vi "HFRR ADV v13.vi"() -> ()   [LabVIEW 2025] (continued)
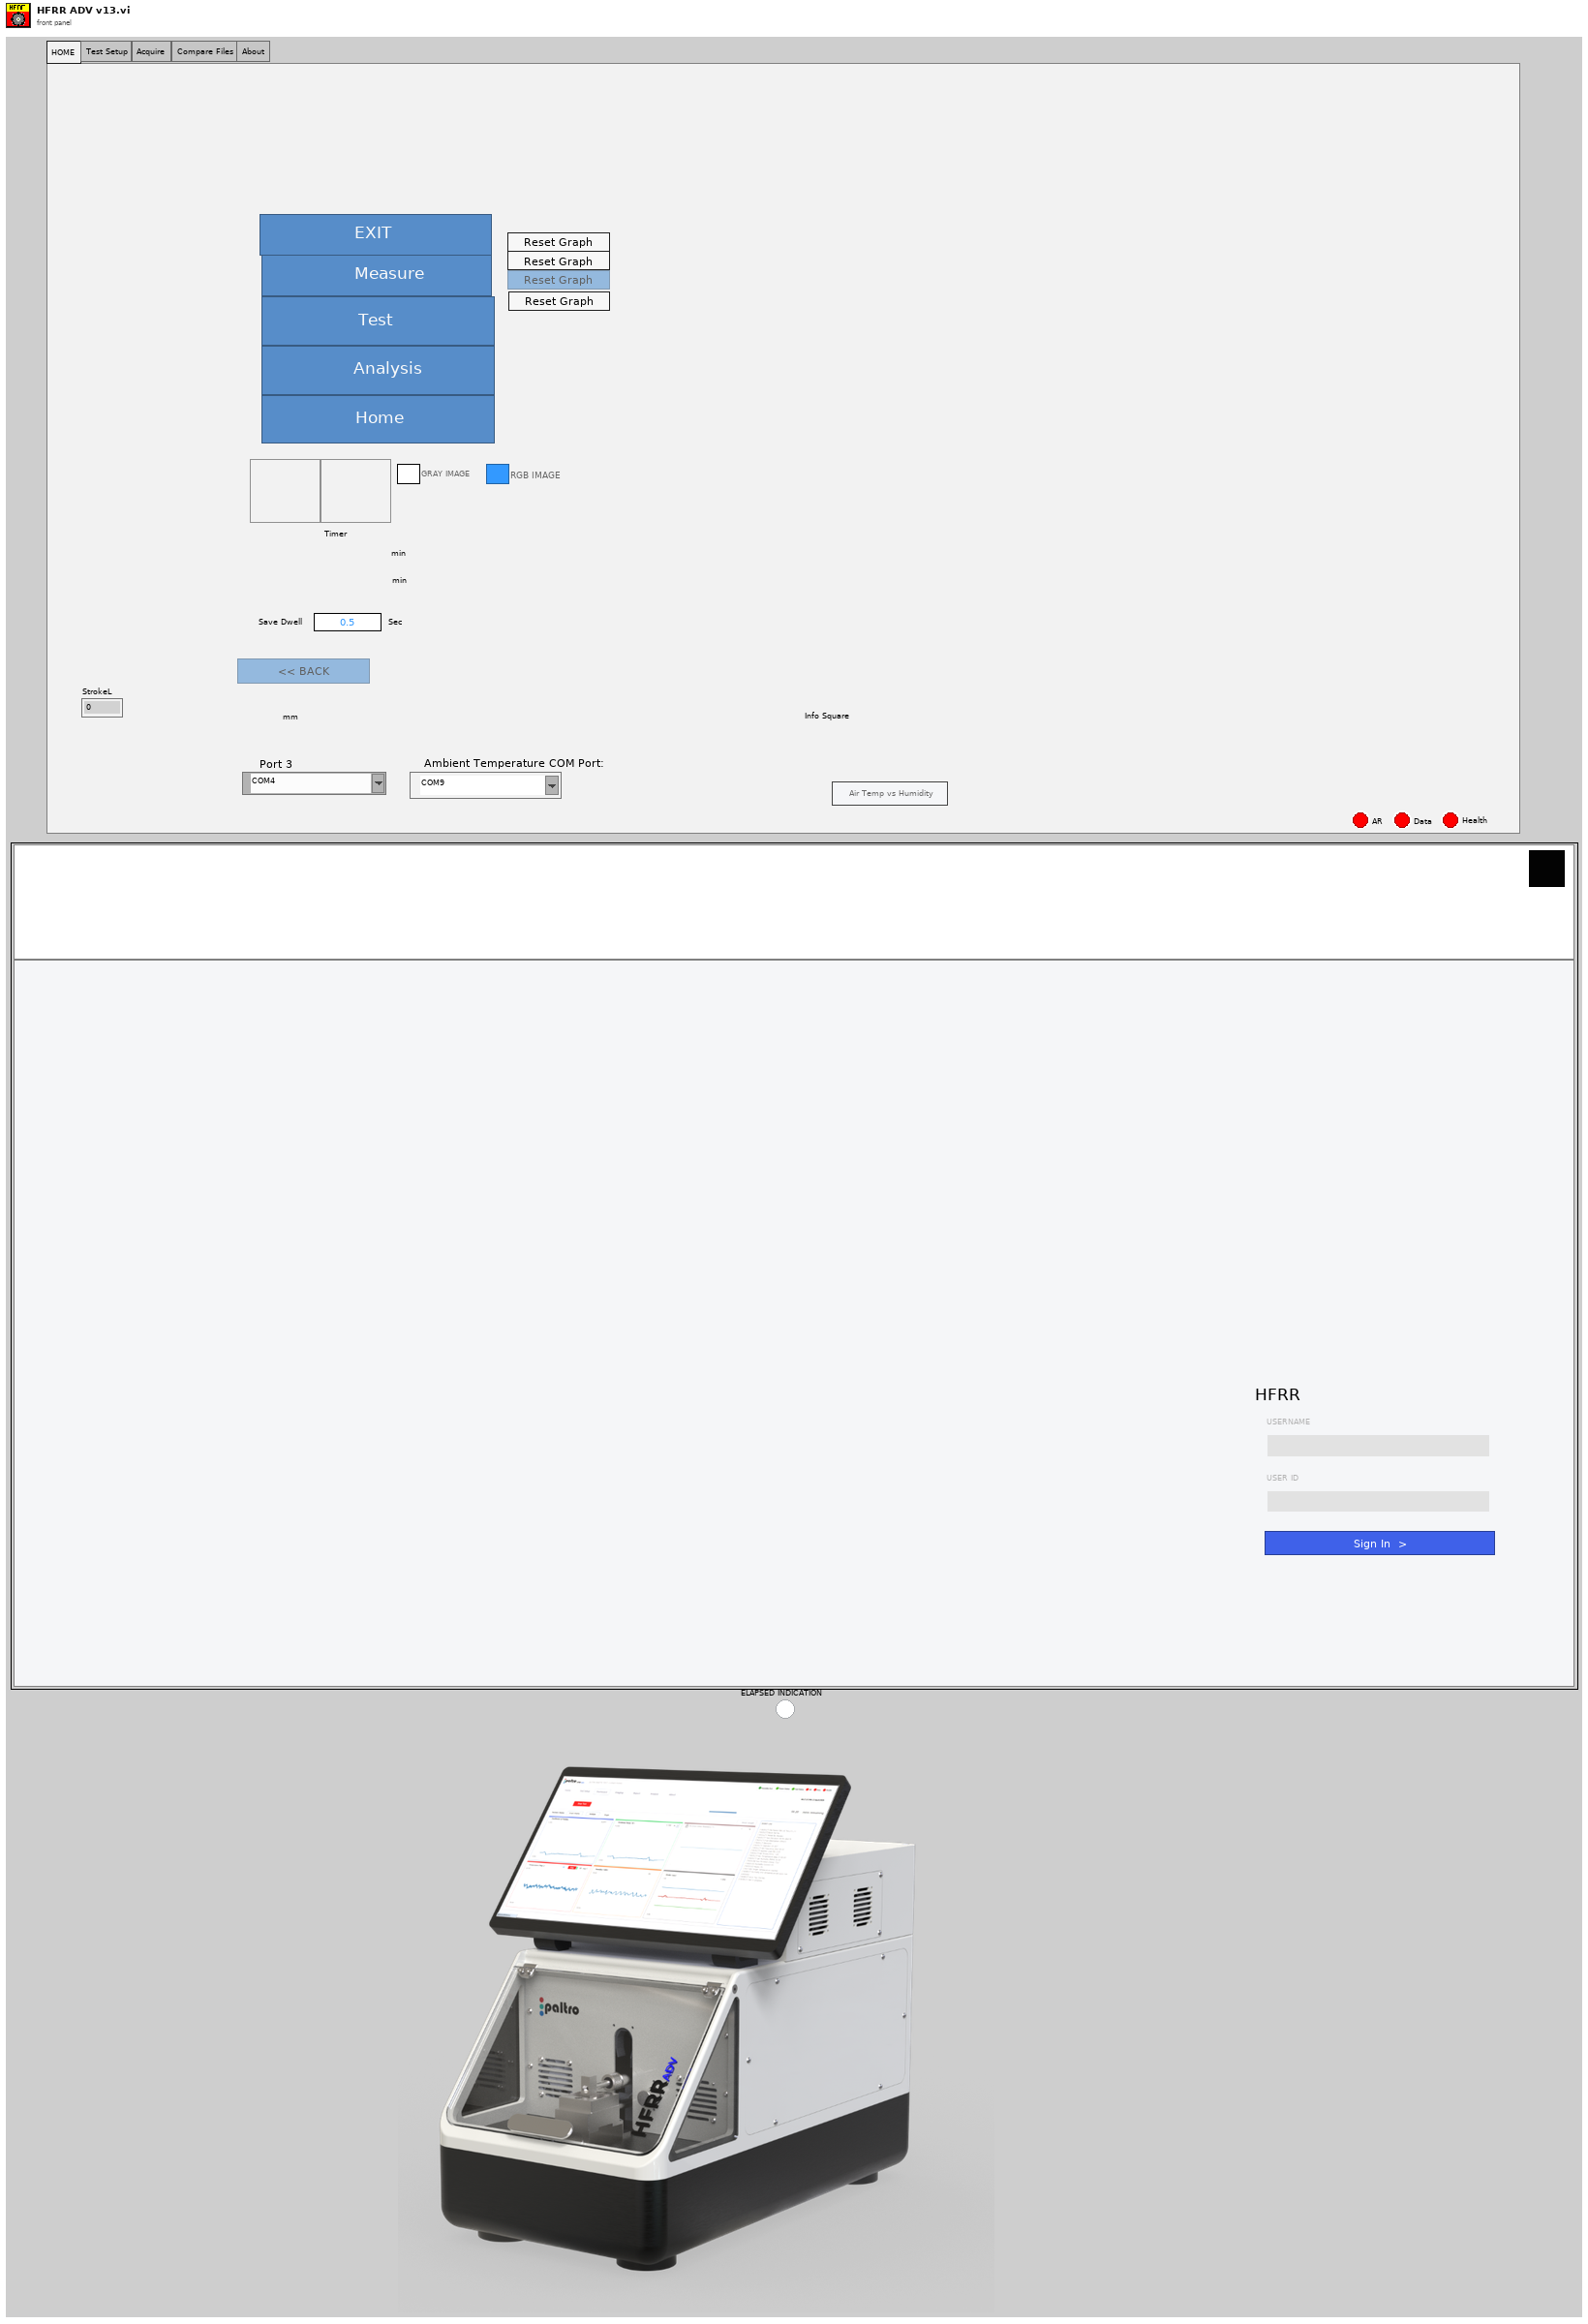
[diagram p1: front panel]
types:
  T1 = enum32{"Home", "Dashboard", "Imaging", "Report", "Analysis", "About", "Test Setup", "Advance"}
  T2 = enum32{"HOME", "Test Setup", "Acquire", "Adv Scar", "Adv Scar Report", "Compare Files", "About", "Advance", "Mooha"}
  T3 = enum16{"ASTM D6079", "ISO 12156", "CEC F-096-A-06", "Custom"}
  T4 = enum32{"Dashboard 1", "Dashboard 2", "Dashboard 3"}
  T5 = enum32{"COF", "Friction", "ECR", "Temperature", "Humidity", "Stroke"}
  T6 = enum32{"Coefficient Of Friction", "Air Temperature", "Humidity", "Stroke", "Sample Temperature", "Electrical Contact Resistance", "Frequency", "Air Temp vs Rh"}
  T7 = enum32{"Gains", "Configuration Parameters", "Temperature Calibration"}
  T8 = enum32{"Stroke Data", "Temperature Calibration", "Friction Force Raw Data"}
  T9 = cluster{"Proportional Gain (Kc)":dbl, "Integral Time (Ti, min)":dbl, "Derivative Time (Td, min)":dbl}
  T10 = enum32{"Temp Variables", "Camera", "WO 2465 (1)", "WO 2465 (2)", "WO 2465 (3)"}
  T11 = typedef "Auto Start enum.ctl" = enum16{"Init", "Humidity & Temperature On", "Reach point", "Maintain Stage", "Start Stage", "close", "Exit"}
  T12 = enum32{"Freqz control", "Low Speed Analog Inputs & Digital IOs", "Temperature Tuning", "Voltage LVDT raw", "High Speed Analog Inputs - Displacement & Friction", "LVDT Calibration", "Sericve", "Friction Force Calibration", "Bytes At Port", "Loadcell Board"}
  T13 = cluster{"proportional gain (Kc)":dbl, "integral time (Ti, min)":dbl, "derivative time (Td, min)":dbl}
  T14 = typedef "imagedata.ctl" = cluster{"image type":i32, "image depth":i32, "image":u8[], "mask":u8[], "colors":u32[], "Rectangle":cluster{"left":i16, "top":i16, "right":i16, "bottom":i16}}
  T15 = enum32{"HOME", "Test Setup", "Acquire", "Compare Files", "Print Report", "About", "Advance", "Mooha"}
  T16 = enum8{"Enabled", "Disabled", "Disabled and Grayed Out"}
  T17 = cluster{"Read Heave and Surge":string, "Bytes at Heave Port":dbl, "Heave and Surge COM Port:":refnum<visa-resource-name>, "Com Port 2":refnum<visa-resource-name>, "Residual Due":string, "Heave COM Status 2":bool, "Heave COM Status":bool, "Port 2":bool, "Sway PPR":dbl, "Surge PPR":dbl, "Heave PPR":dbl, "Sway Pitch":dbl, "Surge Pitch":dbl, "Heave Pitch":dbl, "Sway Pulses/mm":dbl, "Surge Pulses/mm":dbl, "Heave Pulses/mm":dbl, "inner loop":dbl, "Read Heave and Surge 2":string, "String 36":string, "Write S":bool, "WriteCC1":string[], "Heave COM Loop":i32, "LastCom":string, "EXIT":bool, "Error Heave":errorcluster}
  T18 = enum16{"Always On", "Always Off", "Off While Running"}
  T19 = typedef "POST ANALYSIS ENUM.ctl" = enum16{"OPEN EXE", "INIT", "OPEN FILE", "FIT", "DRAW REC", "DRAW LINE", "PAN", "ZOOM IN", "ZOOM OUT", "SET ZOOM", "CLEAR ROI", "GET MEASUREMENTS", "RESIZE MODE", "STREAM START", "STREAM STOP", "SHOW UI", "MINIMIZE UI", "HIDE UI", "CKISE APP", "CLOSE CONNECTION", "SAVE IMAGE", "SET ROI COLOR", "READ", "TCP CHECK", "CLOSE"}
  T20 = typedef "CAMERA LIVE FEED ENUM.ctl" = enum16{"OPEN EXE", "INIT", "READ", "CAMERA CONNECT", "CAMERA START", "CAMERA STOP", "CAMERA GRAY", "CAMERA RGB", "CAMERA MINIMIZE", "CAMERA CLOSE", "CAMERA MODE LIST", "CAMERA MODE SET", "CAMERA RESTORE", "CAMERA SAVE", "CLOSE"}
  T21 = cluster{"File Name":string, "Test Method":string, "Operator":string, "Fuel Description":string, "Date and time":string}
  T22 = enum32{"Home", "Dashboard", "Imaging", "Report", "Analysis", "About", "Test Setup"}
  T23 = enum32{"HOME", "Test Setup", "Acquire", "Compare Files", "About", "Advance", "Mooha"}
  T24 = enum16{"deny read/write", "deny write-only", "deny none"}
  T25 = typedef "NI_ReportGenerationCore.lvlib/HTML Report Image Alignment.ctl" = enum16{"(default)", "LEFT", "RIGHT", "TOP", "TEXTTOP", "MIDDLE", "ABSMIDDLE", "BASELINE", "BOTTOM", "ABSBOTTOM"}
  T26 = enum16{"open", "replace", "create", "open or create", "replace or create", "replace or create with confirmation"}
  T27 = enum16{"INIT", "READ", "MANUAL WRITE", "WRITE", "CLOSE", "ERROR INIT"}
  T28 = enum16{"open", "open or create", "create or replace", "create", "open (read only)"}
  T29 = cluster{"Mode":enum16{"RTU", "ASCII"}, "Slave Address":u8}
diagram:
  w5 = FALSE ("Visible")
  w6 = T16."Enabled" ("Disabled")
  w9 = FALSE ("Visible")
  w8 = FALSE ("Humidity Off Command")
  w28 = "" ("USER ID")
  # "[CH1]    - FF\n[CH2]   - TEMPERATURE\n[CH3]    - Humidity\n[CH4]    - AIR TEMP\n[CH5]\\- Visa Uno\n[CH6] \\- Visa Due\n[CH7]  \\- file path\n[CH8]   - Displacement Gain\n[CHA]   - Stroke Gain\n[CHB]   - Stroke PID Gain\n[CHC]   -Language Selection\n[CHD]   -Power +\n[CHE]   -Power_\n[CHF]   -Heater\n[CHG]   -Humidity Wet\n[CHH]   -Humidity Dry\n[CHI]   -Integral Time \n[CHIJ   -Air intercept\n[CHI]   -Temp Intercept"
  n1 = flat-sequence {
    tunnel: [w83] -> w19
    tunnel: w19 -> [w97]
    tunnel: [w96] -> w18
    tunnel: ["ao0"] -> w21
    tunnel: w18 -> [_]
    tunnel: w21 -> [w162]
    tunnel: [w162] -> w20
    tunnel: w20 -> [w215]
    tunnel: [w213] -> w32
    tunnel: [w215] -> w31
    tunnel: w32 -> [w266]
    tunnel: w31 -> [w222]
    tunnel: [w266] -> w17
    tunnel: [w228] -> w16
    tunnel: [w216] -> w15
    tunnel: [w273] -> _
    tunnel: [w272] -> _
    tunnel: [w274] -> w60
    tunnel: w17 -> [w274]
    tunnel: w16 -> [w272]
    tunnel: w15 -> [w273]
    frame #0 {
      n2 = control-ref of="This VI"() -> (w71:refnum<vi>)
      n3 = property class="VI"(reference=w71) -> (reference out=w62:refnum<vi>, error out=w66:errorcluster, "Panel"=w70:refnum<vi>)  [unwired: 1 in]
      n4 = property class="Pnl"(reference=w70, error in=w66) -> (reference out=w64:refnum<vi>, error out=w67:errorcluster, "Panes[]"=w69:refnum<vi>[])
      n5 = for {
        tunnel: w69 -> [w77] mode=indexing
        tunnel: T18."Always Off" ("Horizontal Scrollbar Visibility") -> [w76]
        tunnel: w67 -> [w73]
        tunnel: [w72] -> w65
        n6 = property class="Pane"(reference=w77, error in=w73, "HorizScrollbarVisibility"=w76) -> (reference out=w74:refnum<vi>, error out=w75:errorcluster)
        n7 = Close Reference(reference=w74, error in (no error)=w75) -> (error out=w72:errorcluster)
      }
      n8 = Close Reference(reference=w64, error in (no error)=w65) -> (error out=w63:errorcluster)
      n9 = Close Reference(reference=w62, error in (no error)=w63) -> (error out=→"error out 8":errorcluster)
    }
    frame #1 {
      n10 = call "CLOSE CONNECTION.vi"("error in (no error)"="error in (no error) 2") -> ("error out"=w81:errorcluster)  [unwired: 10 in]
      n11 = call <vilib>:"Clear Errors.vi"("error in (no error)"=w81) -> ("error out"=w80:errorcluster)  [unwired: 5 in, 1 out]
      n12 = disable-structure shown="Enabled" {
        disable-tunnel: w80 -> [w87 _]
        disable-tunnel: [w86 _] -> w83
        frame Enabled {
          n13 = call <userlib>:"Fit VI window to Largest Dec.vi"("error in (no error)"=w87, "border spacing (2 px)"=1) -> ("error out"=w90:errorcluster, "dup VI Ref"=w94:refnum<vi>)  [unwired: 4 in]
          n14 = invoke on="Invoke Node" class="VI" method="FP.Run-Time Position.Maximized"(reference=w94, error in=w90) -> (error out=w91:errorcluster)  [unwired: 2 in, 3 out]
          n15 = call <vilib>:"Clear Errors.vi"("error in (no error)"=w91) -> ("error out"=w93:errorcluster)  [unwired: 5 in, 1 out]
          n16 = control-ref of="This VI"() -> (w85:refnum<vi>)
          n17 = invoke on="Invoke Node" class="VI" method="Default Vals.Reinit All"(reference=w85, error in=w93) -> (reference out=w89:refnum<vi>, error out=w88:errorcluster)  [unwired: 1 in, 1 out]
          n18 = Close Reference(reference=w89, error in (no error)=w88) -> (error out=w86:errorcluster)
        }
        frame Disabled {
        }
      }
      n19 = local write "sign in temp"(FALSE ("sign in temp")) -> ()
      n20 = property on="Sign In" class="Bool (strict)"("DisabledEnum"=T16."Disabled" ("Disabled")) -> ()  [unwired: 2 in, 2 out]
      n21 = property on="Auto Scar Check" class="Clust (strict)"("Visible"=TRUE) -> ()  [unwired: 2 in, 2 out]
    }
    frame #2 {
      n22 = call "dialog box.vi"("Status"="Before starting the test, verify that the microscope cable is connected.", "error in"=w97) -> ("error out"=w96:errorcluster)  [unwired: 8 in]
    }
    frame #3 {
      w104 = FALSE ("Upld AR 2")
      # "kkkkk"
      # "C:\\Windows\\wndcm_pw_stdED hfrr.txt"
      # "C:\\LAB-IQ NXT"
      # "C:\\LAB-IQ NXT\\wndcm_pw_stdED hfrr.txt"
      # "password file"
      n23 = Current VI's Path() -> (path=w117:path)
      n24 = Strip Path(path=w117) -> (stripped path=w110:path)  [unwired: 1 out]
      n25 = Path To String(path=w110) -> (string=w112:string)
      n26 = local write "conststatus"(0.0 ("rpm value : 2")) -> ()
      n27 = local write "Upld AR 2"(TRUE ("Upld AR 2")) -> ()
      n28 = local write "Lan flag"(0.0 ("Lan flag")) -> ()
      n29 = local write "COUNT"(0 ("COUNT")) -> ()
      n30 = local write "FLAG 2"(0.0 ("FLAG 2")) -> ()
      n31 = local write "Com flag"(u32 0 ("Com flag")) -> ()
      n32 = local write "Re-Initialise"(TRUE ("Re-Initialise")) -> ()
      n33 = local write "refresh flag"(FALSE ("refresh flag")) -> ()
      n34 = local write "Json St Flg"(w104) -> ()
      n35 = Search/Split String(string=w112, search string/char (-)=".exe") -> (match + rest of string=w114:string)  [unwired: 1 in, 2 out]
      n36 = Match True/False String(2:".vi" ("false string"), 3:".exe" ("true string"), 4:w114) -> (0:w111:bool)  [unwired: 1 out]
      n37 = local write "Json End Flg"(w104) -> ()
      n38 = case shown="True" w111 {
        tunnel: w110 -> [w133 w135]
        tunnel: [w133 w134] -> w108
        frame False {
        }
        frame True {
          n39 = Strip Path(path=w135) -> (stripped path=w134:path)  [unwired: 1 out]
        }
      }
      n40 = Path To String(path=w108) -> (string=→"Gain path":string)
      n41 = local write "Main Tab Display"(T4."Dashboard 1" ("Main Tab Display")) -> ()
      n42 = local write "main tab sub"(enum32{"Page 1", "Page 2"}."Page 1" ("main tab sub")) -> ()
      n43 = local write "Main Tab"(T2."HOME" ("Main Tab")) -> ()
      n44 = local write "EVENT LOG"("") -> ()
      n45 = List Folder(path=path "C:/LAB-IQ" ("directory path"), pattern="*.txt") -> (filenames=w123:string[])  [unwired: 2 in, 3 out]
      n46 = Search 1D Array(1D array=w123, element="wndcm_pw_stdED hfrr.txt") -> (index of element=w126:i32)  [unwired: 1 in]
      n47 = Equal?(x=w126, y=-1) -> (x = y?=w121:bool)
      n48 = case shown="True" w121 {
        frame False {
        }
        frame True {
          n49 = String To Byte Array(string="123\n") -> (unsigned byte array=w140:u8[])
          n50 = Array Size(array=w140) -> (size(s)=w139:i32)
          n51 = for {
            N: w139 -> [_]
            tunnel: w140 -> [w153]
            tunnel: [w150] -> w142 mode=indexing
            tunnel: w139 -> [w145]
            i -> [w143]
            n52 = Decrement(x=w145) -> (x-1=w146:i32)
            n53 = Equal?(x=w143, y=w146) -> (x = y?=w147:bool)
            n54 = Index Array(array=w153, index=w143) -> (element=w152:u8)
            n55 = Number To Decimal String(number=w152) -> (decimal integer string=w151:string)  [unwired: 1 in]
            n56 = Select(t="", s=w147, f="\r") -> (s? t:f=w144:string)
            n57 = Concatenate Strings(w151, w144) -> (w150:string)
          }
          n58 = local read "file path"() -> (w136:path)
          n59 = Concatenate Strings(w142) -> (w138:string)
          n60 = call <vilib>:"Write Characters To File.vi"("append to file? (new file:F)"=FALSE, "character string"=w138, "file path (dialog if empty)"=w136) -> ()  [unwired: 2 in, 1 out]
        }
      }
      n61 = local write "clk"(0.0 ("clk")) -> ()
      n62 = local write "Flag"(0.0 ("Flag")) -> ()
      "file path" <- path "C:/LAB-IQ/wndcm_pw_stdED hfrr.txt" ("file path")
      "FF buffer" <- dbl[] [] ("FF buffer")
    }
    frame #4 {
      # "C:\\WinDucom\\calibrate WO 2391.dcf"
      n63 = String To Path(string="C:\\LAB-IQ\\calibrate WO 2465.dcf") -> (path=w161:path)
      n64 = Open/Create/Replace File "Open File"(file path (use dialog)=w161) -> (refnum out=w160:refnum<file>)  [unwired: 5 in, 2 out]
      n65 = for {
        N: 24 -> [_]
        tunnel: w160 -> [w181]
        i -> [w175]
        (unwired) TRUE ("line mode (F)")
        n66 = Read from Text File "Read File"(file (use dialog)=w181) -> (text=w180:string)  [unwired: 3 in, 3 out]
        n67 = Match Pattern(string=w180, regular expression="]") -> (after substring=w178:string)  [unwired: 1 in, 3 out]
        n68 = String Subset(string=w180, offset (0)=5, length (rest)=10 ("length (rest)")) -> (substring=w173:string)
        n69 = Fract/Exp String To Number(string=w173) -> (number=w174:dbl)  [unwired: 3 in, 1 out]
        n70 = Match Pattern(string=w178, regular expression="-") -> (before substring=w176:string)  [unwired: 1 in, 3 out]
        n71 = case shown="7" w175 {
          tunnel: w174 -> [w184 w185 w186 w187 _ _ _ w192 w193 w194 w197 w198 w199 w200 w201 w202 w203 w206 w207 _ _ w210 _ _ _]
          tunnel: w176 -> [_ _ _ _ w188 w189 w190 _ _ _ _ _ _ _ _ _ _ _ _ w208 w209 _ w211 w212 _]
          frame 0 {
            n72 = local write "FRIC. FORCE :"(w184) -> ()
          }
          frame 1 {
            n73 = local write "TEMPERATURE :"(w185) -> ()
          }
          frame 2 {
            n74 = local write "HUMIDITY:"(w186) -> ()
          }
          frame 3 {
            n75 = local write "AIR TEMPERATURE :"(w187) -> ()
          }
          frame 4 {
            n76 = local write "Com Port 1"(w188) -> ()
          }
          frame 5 {
            n77 = local write "Com Port 2"(w189) -> ()
            n78 = local write "visa due"(w189) -> ()
          }
          frame 6 {
            n79 = String To Path(string=w190) -> (path=w191:path)
            n80 = local write "File Path"(w191) -> ()
          }
          frame 7 {
            n81 = local write "DISPLACEMENT :"(w192) -> ()
          }
          frame 8 {
            n82 = local write "STROKE GAIN :"(w193) -> ()
          }
          frame 9 {
            n83 = local read "Stroke PID Gains"() -> (w196:T9)
            n84 = Bundle By Name(cluster=w196, "Proportional Gain (Kc)"=w194) -> (w195:T9)
            n85 = local write "Stroke PID Gains"(w195) -> ()
          }
          frame 10 {
            n86 = local write "Language Selection"(w197) -> ()
          }
          frame 11 {
            n87 = local write "CH-POWER +"(w198) -> ()
          }
          frame 12 {
            n88 = local write "CH-POWER -"(w199) -> ()
          }
          frame 13 {
            n89 = local write "CH-HEATER"(w200) -> ()
          }
          frame 14 {
            n90 = local write "CH-HUMIDITY WET"(w201) -> ()
          }
          frame 15 {
            n91 = local write "CH-HUMIDITY DRY"(w202) -> ()
          }
          frame 16 {
            n92 = local read "Stroke PID Gains"() -> (w205:T9)
            n93 = Bundle By Name(cluster=w205, "Integral Time (Ti, min)"=w203) -> (w204:T9)
            n94 = local write "Stroke PID Gains"(w204) -> ()
          }
          frame 17 {
            n95 = local write "AIR TEMP INTERCEPT:"(w206) -> ()
          }
          frame 18 {
            n96 = local write "TEMP INTERCEPT:"(w207) -> ()
          }
          frame 19 {
            n97 = local write "S.NO"(w208) -> ()
          }
          frame 20 {
            n98 = local write "Com Port 3"(w209) -> ()
          }
          frame 21 {
            n99 = local write "LvdtOff"(w210) -> ()
          }
          frame 22 {
            n100 = local write "C3 :"(w211) -> ()
          }
          frame 23 {
            n101 = local write "Camera Port :"(w212) -> ()
          }
          frame 24, Default {
          }
        }
      }
      n102 = String To Path(string="C:\\LAB-IQ\\Image Calibrate v01.dcf") -> (path=w157:path)
      n103 = Open/Create/Replace File ("Open File")(file path (use dialog)=w157) -> (refnum out=w156:refnum<file>)  [unwired: 5 in, 2 out]
      n104 = for {
        N: 4 -> [_]
        tunnel: w156 -> [w168]
        i -> [w164]
        n105 = Read from Text File ("Read File")(file (use dialog)=w168) -> (text=w169:string)  [unwired: 3 in, 3 out]
        n106 = String Subset(string=w169, offset (0)=6, length (rest)=10 ("length (rest)")) -> (substring=w165:string)
        n107 = Fract/Exp String To Number(string=w165) -> (number=w163:dbl)  [unwired: 3 in, 1 out]
        n108 = case shown="3" w164 {
          tunnel: w163 -> [w170 w171 _ w172 _]
          frame 0 {
            n109 = local write "5x Gain"(w170) -> ()
          }
          frame 1 {
            n110 = local write "10x Gain"(w171) -> ()
          }
          frame 2 {
          }
          frame 3 {
            n111 = local write "100x gain"(w172) -> ()
          }
          frame 4, Default {
          }
        }
      }
    }
    frame #5 {
      n112 = Wait (ms)(milliseconds to wait=u32 1000) -> (millisecond timer value=w213:u32)
    }
    frame #6 {
      w231 = u32 2000 ("milliseconds to wait")
      w258 = u32 2000 ("milliseconds to wait")
      n113 = local read "Re-Initialise"() -> (w265:bool)
      n114 = case shown="True" w265 {
        frame False {
        }
        frame True {
          n115 = local write "Re-Initialise"(FALSE ("Re-Initialise")) -> ()
        }
      }
      n116 = call "CAMERA LIVE FEED FGV.vi"("Enum - Menu"=CAMERA_LIVE_FEED_ENUM."OPEN EXE", "error in (no error)"=w222) -> ("error out"=w264:errorcluster)  [unwired: 8 in, 1 out]
      n117 = call "Stall Data Flow.vim"("value in"=w264, "milliseconds to wait"=w258) -> ("value out"=w262:errorcluster)  [unwired: 1 out]
      n118 = call "CAMERA LIVE FEED FGV.vi"("Enum - Menu"=CAMERA_LIVE_FEED_ENUM."INIT", "error in (no error)"=w262) -> ("error out"=w260:errorcluster)  [unwired: 8 in, 1 out]
      n119 = call "IMAGE ANALYSIS.vi"("Enum"=POST_ANALYSIS_ENUM."OPEN EXE", "error in"=w222) -> ("error out"=w219:errorcluster)  [unwired: 8 in, 1 out]
      n120 = case shown="Error .." w260 {
        selector: w260 -> [w267 _]
        tunnel: [w267 _] -> w259
        frame No Error {
        }
        frame Error {
          n121 = One Button Dialog(message="Camera initialization error.\nPlease Restart the software") -> ()  [unwired: 1 in, 1 out]
        }
      }
      n122 = call "Stall Data Flow.vim"("value in"=w219, "milliseconds to wait"=u32 8000) -> ("value out"=w218:errorcluster)  [unwired: 1 out]
      n123 = property on="Camera Port :" class="CmbBox"() -> ("Strings[]"=w256:string[], "Value"=w257:string)  [unwired: 2 in, 2 out]
      n124 = call "IMAGE ANALYSIS.vi"("Enum"=POST_ANALYSIS_ENUM."INIT", "error in"=w218) -> ("error out"=w216:errorcluster)  [unwired: 8 in, 1 out]
      n125 = Search 1D Array(1D array=w256, element=w257) -> (index of element=w255:i32)  [unwired: 1 in]
      n126 = Type Cast(type=30, x=w255) -> (*(type *) &x=w253:i32)
      n127 = call "Stall Data Flow.vim"("value in"=w259, "milliseconds to wait"=w258) -> ("value out"=w235:errorcluster)  [unwired: 1 out]
      n128 = Add(x=w253, y=48) -> (x+y=w234:i32)
      n129 = call "CAMERA LIVE FEED FGV.vi"("Enum - Menu"=CAMERA_LIVE_FEED_ENUM."CAMERA CONNECT", "error in (no error)"=w235, "CAMERA PORT"=w234) -> ("error out"=w244:errorcluster)  [unwired: 7 in, 1 out]
      n130 = call "Stall Data Flow.vim"("value in"=w244, "milliseconds to wait"=u32 5000) -> ("value out"=w245:errorcluster)  [unwired: 1 out]
      n131 = call "CAMERA LIVE FEED FGV.vi"("Enum - Menu"=CAMERA_LIVE_FEED_ENUM."CAMERA MODE LIST", "error in (no error)"=w245) -> ("error out"=w247:errorcluster)  [unwired: 8 in, 1 out]
      n132 = call "Stall Data Flow.vim"("value in"=w247, "milliseconds to wait"=w231) -> ("value out"=w246:errorcluster)  [unwired: 1 out]
      n133 = call "CAMERA LIVE FEED FGV.vi"("Enum - Menu"=CAMERA_LIVE_FEED_ENUM."READ", "error in (no error)"=w246) -> ("error out"=w233:errorcluster, "data out"=→"Camera List":string)  [unwired: 8 in]
      n134 = call "Stall Data Flow.vim"("value in"=w233, "milliseconds to wait"=w231) -> ("value out"=w232:errorcluster)  [unwired: 1 out]
      n135 = Type Cast(type=30, x=0) -> (*(type *) &x=w227:i32)
      n136 = Add(x=w227, y=48) -> (x+y=w225:i32)
      n137 = call "CAMERA LIVE FEED FGV.vi"("Enum - Menu"=CAMERA_LIVE_FEED_ENUM."CAMERA MODE SET", "error in (no error)"=w232, "CAMERA MODE"=w225) -> ("error out"=w229:errorcluster)  [unwired: 7 in, 1 out]
      n138 = call "Stall Data Flow.vim"("value in"=w229, "milliseconds to wait"=u32 2000) -> ("value out"=w249:errorcluster)  [unwired: 1 out]
      n139 = call "CAMERA LIVE FEED FGV.vi"("Enum - Menu"=CAMERA_LIVE_FEED_ENUM."CAMERA START", "error in (no error)"=w249) -> ("error out"=w250:errorcluster)  [unwired: 8 in, 1 out]
      n140 = call "Stall Data Flow.vim"("value in"=w250, "milliseconds to wait"=u32 1000) -> ("value out"=w251:errorcluster)  [unwired: 1 out]
      n141 = call "CAMERA LIVE FEED FGV.vi"("Enum - Menu"=CAMERA_LIVE_FEED_ENUM."CAMERA MINIMIZE", "error in (no error)"=w251) -> ("error out"=w228:errorcluster)  [unwired: 8 in, 1 out]
    }
    frame #7 {
      n142 = case shown="No Error" w272 {
        frame No Error {
          n143 = property on="Auto Scar Check" class="Clust (strict)"("Visible"=FALSE) -> ()  [unwired: 2 in, 2 out]
        }
        frame Error {
        }
      }
      n144 = local write "sign in temp"(TRUE ("sign in temp")) -> ()
      n145 = property on="Sign In" class="Bool (strict)"("DisabledEnum"=T16."Enabled" ("Disabled")) -> ()  [unwired: 2 in, 2 out]
    }
  }
  n146 = local write "Cal Password"("" ("Cal Password")) -> ()
  n147 = property on="Auto Start Test" class="Bool (strict)"("Visible"=TRUE) -> ()  [unwired: 2 in, 2 out]
  n148 = property on="FRICVALZ 2" class="Bool (strict)"("DisabledEnum"=w6) -> ()  [unwired: 2 in, 2 out]
  n149 = property on="FRICVALZ 4" class="Bool (strict)"("DisabledEnum"=w6) -> ()  [unwired: 2 in, 2 out]
  n150 = property on="FRICVALZ 3" class="Bool (strict)"("DisabledEnum"=w6) -> ()  [unwired: 2 in, 2 out]
  n151 = property on="About" class="Clust (strict)"("Visible"=FALSE) -> ()  [unwired: 2 in, 2 out]
  n152 = property on="Tab Control 5" class="TabCtl (strict)"("Tabs Visible?"=TRUE ("Page Labels Display Visible?")) -> ()  [unwired: 2 in, 2 out]
  n153 = property on="Wrong Password" class="Str"("Visible"=w5) -> ()  [unwired: 2 in, 2 out]
  n154 = property on="Calibration 2" class="TabCtl (strict)"("Visible"=w5) -> ()  [unwired: 2 in, 2 out]
  n155 = local write "SCAR MEASURMENT"(enum32{"Auto Scar", "Manual Scar"}."Manual Scar" ("SCAR MEASURMENT")) -> ()
  n156 = local write "Temperature Off Command"(w8) -> ()
  n157 = local write "Main Dashboard Buttons"(T1."Home" ("Main Dashboard Buttons")) -> ()
  n158 = local write "Humidity Off Command"(w8) -> ()
  n159 = local write "CAMERA ROI MIN TEMP"(w8) -> ()
  n160 = local write "TEST FILE NAM,E SAVED"(w8) -> ()
  n161 = local write "LIVE FEED MIN TEMP"(w8) -> ()
  n162 = local write "SCAR MEASURMENT"(enum32{"Auto Scar", "Manual Scar"}."Manual Scar" ("SCAR MEASURMENT")) -> ()
  n163 = while {
    stop <- w276 stop-if-true
    n164 = event shown="[1] \"RUN\": Value Change" {
      selector: _ -> [_ _ _ _ _ _ _ _ _ _ _ _ _]
      dyn-events: _ -> [_ _ _ _ _ _ _ _ _ _ _ _ _]
      timeout: 100 -> [_ _ _ _ _ _ _ _ _ _ _ _ _]
      tunnel: [FALSE FALSE _ FALSE _ _ _ _ _ _ _ _ TRUE] -> w276
      event Timeout {
        n165 = event-data() -> ()  [unwired: 1 in, 3 out]
        n166 = local read "Auto Start Test"() -> (w280:bool)
        n167 = local read "RUN"() -> (w281:bool)
        n168 = Or(x=w281, y=w280) -> (x .or. y?=w279:bool)
        n169 = case shown="True" w279 {
          frame False {
            w292 = TRUE ("PAUSE")
            n170 = call "ELAPSED TIMER VI - abort test.vi"("RESET"=w292, "PAUSE"=w292) -> ()  [unwired: 7 in, 3 out]
          }
          frame True {
            n171 = local read "Stroke 2"() -> (w297:dbl)
            n172 = local read "FF 3"() -> (w299:dbl)
            n173 = Equal?(x=w297, y=0.95 ("Stroke 2")) -> (x = y?=w294:bool)
            n174 = Equal?(x=w299, y=0.0 ("FF 3")) -> (x = y?=w295:bool)
            n175 = Or(x=w295, y=w294) -> (x .or. y?=w293:bool)
            n176 = case shown="True" w293 {
              selector: w293 -> [_ w304]
              frame False {
                w300 = TRUE ("PAUSE")
                n177 = call "ELAPSED TIMER VI - abort test.vi"("RESET"=w300, "PAUSE"=w300) -> ()  [unwired: 7 in, 3 out]
              }
              frame True {
                n178 = Not(x=w304) -> (.not. x?=w303:bool)
                n179 = call "ELAPSED TIMER VI - abort test.vi"("TARGET"=60.0, "RESET"=w303, "PAUSE"=FALSE) -> ("ELAPSED INDICATION"=w301:bool)  [unwired: 6 in, 2 out]
                n180 = case shown="True" w301 {
                  frame False {
                  }
                  frame True {
                    n181 = stacked-sequence {
                      frame #0 {
                        w306 = FALSE
                        n182 = local write "RUN"(w306) -> ()
                        n183 = local write "Auto Start Test"(w306) -> ()
                      }
                      frame #1 {
                        n184 = One Button Dialog(message="Test stopped due to a communication error. Reconnect the C1 and C2 cables.") -> ()  [unwired: 1 in, 1 out]
                      }
                    }
                  }
                }
              }
            }
          }
        }
        n185 = Get Date/Time In Seconds() -> (seconds since 1Jan1904=w290:timestamp)
        n186 = Format Into String(format string="%<%I:%M:%S:%p %d:%B:%Y>T", w290) -> (resulting string=→"Time Stamp":string)  [unwired: 2 in, 1 out]
        n187 = local read "Service Password enable"() -> (w282:bool)
        n188 = local read "FILE"() -> (w287:string)
        n189 = call <vilib>:"Trim Whitespace.vi"("string"=w287) -> ("trimmed string"=w286:string)  [unwired: 1 in]
        n190 = String Length(string=w286) -> (length=w285:i32)
        n191 = Greater?(x=w285, y=1) -> (0:w283:bool)
        n192 = case shown="False" w283 {
          tunnel: w282 -> [w308 _]
          frame False {
            n193 = case shown="True" w308 {
              frame True {
                w309 = "Test Start In Service Mode" ("Tip Strip")
                w310 = T16."Enabled" ("Disabled")
                n194 = property on="Auto Start Test" class="Bool (strict)"("DisabledEnum"=w310, "TipStrip"=w309) -> ()  [unwired: 2 in, 2 out]
                n195 = property on="RUN" class="Bool (strict)"("DisabledEnum"=w310, "TipStrip"=w309) -> ()  [unwired: 2 in, 2 out]
              }
              frame False {
                w311 = "Enter File Name to Start Test" ("Tip Strip")
                w312 = T16."Disabled and Grayed Out" ("Disabled")
                n196 = property on="Auto Start Test" class="Bool (strict)"("DisabledEnum"=w312, "TipStrip"=w311) -> ()  [unwired: 2 in, 2 out]
                n197 = property on="RUN" class="Bool (strict)"("DisabledEnum"=w312, "TipStrip"=w311) -> ()  [unwired: 2 in, 2 out]
              }
            }
          }
          frame True {
            w313 = "" ("Tip Strip")
            w314 = T16."Enabled" ("Disabled")
            n198 = property on="Auto Start Test" class="Bool (strict)"("DisabledEnum"=w314, "TipStrip"=w313) -> ()  [unwired: 2 in, 2 out]
            n199 = property on="RUN" class="Bool (strict)"("DisabledEnum"=w314, "TipStrip"=w313) -> ()  [unwired: 2 in, 2 out]
          }
        }
      }
      event "RUN": Value Change {
        n200 = event-data() -> ()  [unwired: 1 in, 6 out]
        n201 = local read "RUN"() -> (w316:bool)
        n202 = case shown="True" w316 {
          frame False {
            w317 = T16."Enabled" ("Disabled")
            w321 = "" ("FILE")
            n203 = local write "FILE"(w321) -> ()
            n204 = local write "Batch Ref Num :"(w321) -> ()
            n205 = local write "Fuel Discription :"(w321) -> ()
            n206 = local write "Main Tab"(T2."Adv Scar" ("Main Tab")) -> ()
            n207 = local write "Remarks :"(w321) -> ()
            n208 = local write "Main Dashboard Buttons"(T1."Imaging" ("Main Dashboard Buttons")) -> ()
            n209 = local write "TEST FILE NAM,E SAVED"(FALSE ("TEST FILE NAM,E SAVED")) -> ()
            n210 = property on="Stroke ( mm )" class="WFChart (strict)"("History Data"=cluster{"y":dbl, dbl, "y":dbl}[] []) -> ()  [unwired: 2 in, 2 out]
            n211 = property on="Auto Start Test" class="Bool (strict)"("Visible"=TRUE) -> ()  [unwired: 2 in, 2 out]
            n212 = property on="FRICVALZ 2" class="Bool (strict)"("DisabledEnum"=w317) -> ()  [unwired: 2 in, 2 out]
            n213 = property on="FRICVALZ 4" class="Bool (strict)"("DisabledEnum"=w317) -> ()  [unwired: 2 in, 2 out]
            n214 = property on="FRICVALZ 3" class="Bool (strict)"("DisabledEnum"=w317) -> ()  [unwired: 2 in, 2 out]
          }
          frame True {
            w324 = T16."Disabled" ("Disabled")
            n215 = property on="Auto Start Test" class="Bool (strict)"("Visible"=FALSE) -> ()  [unwired: 2 in, 2 out]
            n216 = property on="FRICVALZ 2" class="Bool (strict)"("DisabledEnum"=w324) -> ()  [unwired: 2 in, 2 out]
            n217 = property on="FRICVALZ 4" class="Bool (strict)"("DisabledEnum"=w324) -> ()  [unwired: 2 in, 2 out]
            n218 = property on="FRICVALZ 3" class="Bool (strict)"("DisabledEnum"=w324) -> ()  [unwired: 2 in, 2 out]
          }
        }
      }
      event "Auto": Value Change {
        n219 = event-data() -> ()  [unwired: 1 in, 6 out]
        n220 = stacked-sequence {
          frame #0 {
            n221 = local write "FILE"("") -> ()
          }
          frame #1 {
            n222 = Get Date/Time In Seconds() -> (seconds since 1Jan1904=w330:timestamp)
            n223 = Format Into String(format string="%<%I_%M_%S_%p_%d_%B_%Y>T", w330) -> (resulting string=w329:string)  [unwired: 2 in, 1 out]
            n224 = local write "FILE"(w329) -> ()
          }
        }
        n225 = local read "Auto"() -> (w327:bool)
        n226 = Not(x=w327) -> (.not. x?=w326:bool)
        n227 = local write "Auto"(w326) -> ()
      }
      event "Auto Start Test": Value Change {
        n228 = event-data() -> ()  [unwired: 1 in, 6 out]
        n229 = local read "Auto Start Test"() -> (w333:bool)
        n230 = case shown="True" w333 {
          frame False {
            w334 = T16."Enabled" ("Disabled")
            w338 = "" ("FILE")
            n231 = local write "Main Tab"(T2."Adv Scar" ("Main Tab")) -> ()
            n232 = local write "Main Dashboard Buttons"(T1."Imaging" ("Main Dashboard Buttons")) -> ()
            n233 = property on="RUN" class="Bool (strict)"("Visible"=TRUE) -> ()  [unwired: 2 in, 2 out]
            n234 = local write "TEST FILE NAM,E SAVED"(FALSE ("TEST FILE NAM,E SAVED")) -> ()
            n235 = local write "Fuel Discription :"(w338) -> ()
            n236 = local write "Batch Ref Num :"(w338) -> ()
            n237 = local write "Remarks :"(w338) -> ()
            n238 = local write "FILE"(w338) -> ()
            n239 = property on="FRICVALZ 2" class="Bool (strict)"("DisabledEnum"=w334) -> ()  [unwired: 2 in, 2 out]
            n240 = property on="FRICVALZ 4" class="Bool (strict)"("DisabledEnum"=w334) -> ()  [unwired: 2 in, 2 out]
            n241 = property on="FRICVALZ 3" class="Bool (strict)"("DisabledEnum"=w334) -> ()  [unwired: 2 in, 2 out]
          }
          frame True {
            w340 = T16."Disabled" ("Disabled")
            n242 = property on="RUN" class="Bool (strict)"("Visible"=FALSE) -> ()  [unwired: 2 in, 2 out]
            n243 = property on="FRICVALZ 2" class="Bool (strict)"("DisabledEnum"=w340) -> ()  [unwired: 2 in, 2 out]
            n244 = property on="FRICVALZ 4" class="Bool (strict)"("DisabledEnum"=w340) -> ()  [unwired: 2 in, 2 out]
            n245 = property on="FRICVALZ 3" class="Bool (strict)"("DisabledEnum"=w340) -> ()  [unwired: 2 in, 2 out]
          }
        }
      }
      event "FILE", "USERNAME", "USER ID": Mouse Enter {
        n246 = event-data() -> ()  [unwired: 1 in, 4 out]
        n247 = dll-call lib="kernel32.dll" fn="Wow64DisableWow64FsRedirection"("OldValue"=0) -> (error out=w347:errorcluster, "OldValue"=w345:i32)  [unwired: 4 in, 1 out]
        n248 = call <vilib>:"System Exec.vi"("run minimized? (F)"=TRUE, "error in (no error)"=w347, "command line"="C:\\Program Files\\Common Files\\Microsoft Shared\\Ink\\TabTip.exe") -> ("error out"=w346:errorcluster)  [unwired: 5 in, 3 out]
        n249 = dll-call lib="kernel32.dll" fn="Wow64EnableWow64FsRedirection"(error in=w346, "OldValue"=w345) -> ()  [unwired: 4 in, 2 out]
      }
      event "EDIT": Value Change {
        n250 = event-data() -> ()  [unwired: 1 in, 6 out]
        n251 = local read "EDIT"() -> (w348:bool)
        n252 = case shown="False" w348 {
          frame False {
            n253 = control-ref of="This VI"() -> (w365:refnum<vi>)
            n254 = property class="VI"(reference=w365) -> (reference out=w356:refnum<vi>, error out=w360:errorcluster, "Panel"=w364:refnum<vi>)  [unwired: 1 in]
            n255 = property class="Pnl"(reference=w364, error in=w360) -> (reference out=w358:refnum<vi>, error out=w361:errorcluster, "Panes[]"=w363:refnum<vi>[])
            n256 = for {
              tunnel: w363 -> [w371] mode=indexing
              tunnel: T18."Always Off" ("Horizontal Scrollbar Visibility") -> [w370]
              tunnel: w361 -> [w367]
              tunnel: [w366] -> w359
              n257 = property class="Pane"(reference=w371, error in=w367, "HorizScrollbarVisibility"=w370) -> (reference out=w368:refnum<vi>, error out=w369:errorcluster)
              n258 = Close Reference(reference=w368, error in (no error)=w369) -> (error out=w366:errorcluster)
            }
            n259 = Close Reference(reference=w358, error in (no error)=w359) -> (error out=w357:errorcluster)
            n260 = Close Reference(reference=w356, error in (no error)=w357) -> (error out=w351:errorcluster)
            "error out 7" <- w351
            n261 = call <vilib>:"Clear Errors.vi"("error in (no error)"=w351) -> ("error out"=w350:errorcluster)  [unwired: 5 in, 1 out]
            n262 = local write "Service Password enable"(FALSE ("Service Password enable")) -> ()
            n263 = call <userlib>:"Fit VI window to Largest Dec.vi"("error in (no error)"=w350, "border spacing (2 px)"=1) -> ("error out"=w355:errorcluster, "dup VI Ref"=w353:refnum<vi>)  [unwired: 4 in]
            n264 = invoke on="Invoke Node" class="VI" method="FP.Run-Time Position.Maximized"(reference=w353, error in=w355) -> (error out=w354:errorcluster)  [unwired: 2 in, 3 out]
            n265 = call <vilib>:"Clear Errors.vi"("error in (no error)"=w354) -> ()  [unwired: 5 in, 2 out]
          }
          frame True {
          }
        }
      }
      event "Headen Service Button": Value Change {
        n266 = event-data() -> ()  [unwired: 1 in, 6 out]
        n267 = local read "Headen Service Button"() -> (w372:bool)
        n268 = case shown="True" w372 {
          frame False {
            n269 = property on="Password 3" class="Clust (strict)"("Visible"=FALSE) -> ()  [unwired: 2 in, 2 out]
            n270 = property on="Service Password Log" class="Str"("Visible"=FALSE) -> ()  [unwired: 2 in, 2 out]
          }
          frame True {
            n271 = property on="Password 3" class="Clust (strict)"("Visible"=TRUE) -> ()  [unwired: 2 in, 2 out]
            n272 = property on="Service Password Log" class="Str"("Visible"=TRUE) -> ()  [unwired: 2 in, 2 out]
          }
        }
      }
      event "Password 3.Service Password": Value Change {
        n273 = event-data() -> ()  [unwired: 1 in, 6 out]
        n274 = Unbundle By Name("Password 3") -> ("Service Password"=w379:string)
        n275 = call <vilib>:"Trim Whitespace.vi"("string"=w379) -> ("trimmed string"=w377:string)  [unwired: 1 in]
        n276 = Equal?(x=w377, y="Service@123") -> (x = y?=w378:bool)
        n277 = case shown="False" w378 {
          selector: w378 -> [w383 w385]
          frame False {
            n278 = local write "Service Password enable"(w383) -> ()
            n279 = property on="Service Password Log" class="Str"("Visible"=TRUE) -> ()  [unwired: 2 in, 2 out]
            n280 = property on="Tab Control 5" class="TabCtl (strict)"("Tabs Visible?"=TRUE ("Page Labels Display Visible?")) -> ()  [unwired: 2 in, 2 out]
          }
          frame True {
            n281 = property on="Service Password Log" class="Str"("Visible"=FALSE) -> ()  [unwired: 2 in, 2 out]
            "Service Password enable" <- w385
          }
        }
      }
      event "Sign In": Value Change {
        w387 = FALSE ("Visible")
        n282 = event-data() -> ()  [unwired: 1 in, 6 out]
        n283 = property on="About" class="Clust (strict)"("Visible"=w387) -> ()  [unwired: 2 in, 2 out]
        n284 = property on="Password 3" class="Clust (strict)"("Visible"=w387) -> ()  [unwired: 2 in, 2 out]
        n285 = property on="Service Password Log" class="Str"("Visible"=FALSE) -> ()  [unwired: 2 in, 2 out]
      }
      event "Info": Value Change {
        n286 = event-data() -> ()  [unwired: 1 in, 6 out]
        n287 = local read "Info"() -> (w389:bool)
        n288 = case shown="False" w389 {
          frame False {
            n289 = property on="About" class="Clust (strict)"("Visible"=FALSE) -> ()  [unwired: 2 in, 2 out]
          }
          frame True {
            n290 = property on="About" class="Clust (strict)"("Visible"=TRUE) -> ()  [unwired: 2 in, 2 out]
          }
        }
      }
      event "Calibration": Value Change {
        n291 = event-data() -> ()  [unwired: 1 in, 6 out]
        n292 = local read "Calibration"() -> (w393:bool)
        n293 = case shown="False" w393 {
          frame False {
            n294 = property on="Calibration 2" class="TabCtl (strict)"("Visible"=FALSE) -> ()  [unwired: 2 in, 2 out]
            n295 = local write "Cal Password"("" ("Cal Password")) -> ()
          }
          frame True {
            n296 = property on="Calibration 2" class="TabCtl (strict)"("Visible"=TRUE) -> ()  [unwired: 2 in, 2 out]
            n297 = local write "Cal Password"("" ("Cal Password")) -> ()
          }
        }
        n298 = property on="Wrong Password" class="Str"("Visible"=FALSE) -> ()  [unwired: 2 in, 2 out]
      }
      event "Cal Password": Value Change {
        n299 = event-data() -> ()  [unwired: 1 in, 6 out]
        n300 = local read "Cal Password"() -> (w401:string)
        n301 = call <vilib>:"Trim Whitespace.vi"("string"=w401) -> ("trimmed string"=w400:string)  [unwired: 1 in]
        n302 = Equal?(x=w400, y="Cal@321") -> (x = y?=w398:bool)
        n303 = case shown="True" w398 {
          frame False {
            n304 = property on="Wrong Password" class="Str"("Visible"=TRUE) -> ()  [unwired: 2 in, 2 out]
          }
          frame True {
            n305 = property on="Wrong Password" class="Str"("Visible"=FALSE) -> ()  [unwired: 2 in, 2 out]
            n306 = local write "Main Tab"(T2."About" ("Main Tab")) -> ()
            n307 = local write "Cal Password"("" ("Cal Password")) -> ()
            n308 = local write "Main Dashboard Buttons"(T1."About" ("Main Dashboard Buttons")) -> ()
            n309 = local write "Tab Control 5"(T7."Temperature Calibration" ("Tab Control 5")) -> ()
            n310 = property on="Calibration 2" class="TabCtl (strict)"("Visible"=FALSE) -> ()  [unwired: 2 in, 2 out]
            n311 = property on="Tab Control 5" class="TabCtl (strict)"("Tabs Visible?"=FALSE ("Page Labels Display Visible?")) -> ()  [unwired: 2 in, 2 out]
            n312 = local write "Calibration"(FALSE ("Calibration")) -> ()
          }
        }
      }
      event "Quit": Value Change {
        n313 = event-data() -> ()  [unwired: 1 in, 6 out]
      }
    }
    n314 = Wait (ms)(milliseconds to wait=u32 100) -> ()  [unwired: 1 out]
  }
  n315 = local write "Auto stop temp"(w9) -> ()
  n316 = local write "main tab sub"(enum32{"Page 1", "Page 2"}."Page 1" ("main tab sub")) -> ()
  n317 = local write "USERNAME"(w28) -> ()
  n318 = local write "Main Tab"(T2."HOME" ("Main Tab")) -> ()
  n319 = local write "USER ID"(w28) -> ()
  n320 = property on="Auto Scar Check  2" class="Clust (strict)"("Visible"=w9) -> (error out=w13:errorcluster)  [unwired: 2 in, 1 out]
  n321 = property on="Quit" class="Bool (strict)"("Value"=FALSE ("Quit")) -> (error out=w30:errorcluster)  [unwired: 2 in, 1 out]
  n322 = while {
    shift-right: [w413] -> _
    shift-left: "Enum - Selector" -> [w414]
    stop <- w415 stop-if-true
    # "Auto Start Logic Loop"
    n323 = case shown="\"close\"" w414 {
      tunnel: [w418 w424 w435 w467 w498 Auto_Start_enum."Exit" ("Enum - Selector") Auto_Start_enum."Init" ("Enum - Selector")] -> w413
      frame "Init", Default {
        n324 = local read "Auto Start Test"() -> (w417:bool)
        n325 = Select(t=Auto_Start_enum."Humidity & Temperature On" ("Enum - Selector"), s=w417, f=Auto_Start_enum."Init") -> (s? t:f=w418:T11)
      }
      frame "Humidity & Temperature On" {
        n326 = flat-sequence {
          tunnel: [Auto_Start_enum."Reach point" ("Enum - Selector")] -> w421
          frame #0 {
            w425 = T16."Disabled and Grayed Out" ("Disabled")
            w426 = TRUE ("Heater Button")
            n327 = property on="Humidity" class="Bool (strict)"("DisabledEnum"=w425) -> ()  [unwired: 2 in, 2 out]
            n328 = property on="Heater Button" class="Bool (strict)"("DisabledEnum"=w425) -> ()  [unwired: 2 in, 2 out]
            n329 = local write "Heater Button"(w426) -> ()
            n330 = local write "Humidity"(w426) -> ()
          }
          frame #1 {
            n331 = Wait (ms)(milliseconds to wait=u32 1000) -> ()  [unwired: 1 out]
          }
          frame #2 {
            w428 = TRUE ("Reach point temp")
            n332 = local write "Reach point Humidity"(w428) -> ()
            n333 = local write "Reach point temp"(w428) -> ()
          }
        }
        n334 = local read "Auto Start Test"() -> (w423:bool)
        n335 = Not(x=w423) -> (.not. x?=w422:bool)
        n336 = Select(t=Auto_Start_enum."close", s=w422, f=w421) -> (s? t:f=w424:T11)
      }
      frame "Reach point" {
        w436 = TRUE ("PAUSE")
        w444 = 1.0 ("y")
        w447 = 1.0 ("y")
        n337 = local read "Set Temperature:"() -> (w448:dbl)
        n338 = local read "Set Humidity:"() -> (w443:dbl)
        n339 = local read "Humidity ( %RH )"() -> (w449:dbl)
        n340 = Add(x=w448, y=w447) -> (x+y=w446:dbl)
        n341 = Subtract(x=w448, y=w447) -> (x-y=w445:dbl)
        n342 = Add(x=w443, y=w444) -> (x+y=w442:dbl)
        n343 = Subtract(x=w443, y=w444) -> (x-y=w441:dbl)
        n344 = local read "TEMP"() -> (w450:dbl)
        n345 = In Range and Coerce(upper limit=w442, x=w449, lower limit=w441) -> (In Range?=w430:bool)  [unwired: 1 out]
        n346 = In Range and Coerce(upper limit=w446, x=w450, lower limit=w445) -> (In Range?=w431:bool)  [unwired: 1 out]
        n347 = case shown="True" w430 {
          frame False {
          }
          frame True {
            n348 = case shown="True" "Reach point Humidity" {
              selector: "Reach point Humidity" -> [_ w456]
              frame False {
              }
              frame True {
                n349 = local read "EVENT LOG"() -> (w453:string)
                n350 = Not(x=w456) -> (.not. x?=w455:bool)
                n351 = local write "Reach point Humidity"(w455) -> ()
                n352 = call "Event Log.vi"("Content"="Target Humidity reached", "EVENT LOG"=w453) -> ("EVENT LOG"=w454:string)  [unwired: 8 in, 1 out]
                n353 = local write "EVENT LOG"(w454) -> ()
              }
            }
          }
        }
        n354 = case shown="True" w431 {
          frame False {
          }
          frame True {
            n355 = case shown="True" "Reach point temp" {
              selector: "Reach point temp" -> [_ w462]
              frame False {
              }
              frame True {
                n356 = local read "EVENT LOG"() -> (w459:string)
                n357 = Not(x=w462) -> (.not. x?=w461:bool)
                n358 = local write "Reach point temp"(w461) -> ()
                n359 = call "Event Log.vi"("Content"="Target Temperature reached", "EVENT LOG"=w459) -> ("EVENT LOG"=w460:string)  [unwired: 8 in, 1 out]
                n360 = local write "EVENT LOG"(w460) -> ()
              }
            }
          }
        }
        n361 = local read "Auto Start Test"() -> (w434:bool)
        n362 = And(x=w431, y=w430) -> (x .and. y?=w440:bool)
        n363 = Select(t=Auto_Start_enum."Maintain Stage" ("Enum - Selector"), s=w440, f=Auto_Start_enum."Reach point" ("Enum - Selector")) -> (s? t:f=w437:T11)
        n364 = Not(x=w434) -> (.not. x?=w433:bool)
        n365 = Select(t=Auto_Start_enum."close", s=w433, f=w437) -> (s? t:f=w435:T11)
        n366 = call "ELAPSED TIMER VI.vi"("RESET"=w436, "PAUSE"=w436) -> ()  [unwired: 7 in, 3 out]
      }
      frame "Maintain Stage" {
        w476 = 2.0 ("y")
        w475 = 1.0 ("y")
        # "Humidity and  temperatures Set Point  have been reached"
        n367 = local read "Set Temperature:"() -> (w482:dbl)
        n368 = local read "Set Humidity:"() -> (w479:dbl)
        n369 = local read "Humidity ( %RH )"() -> (w483:dbl)
        n370 = Add(x=w482, y=w475) -> (x+y=w481:dbl)
        n371 = Subtract(x=w482, y=w475) -> (x-y=w480:dbl)
        n372 = local read "TEMP"() -> (w484:dbl)
        n373 = Add(x=w479, y=w476) -> (x+y=w478:dbl)
        n374 = Subtract(x=w479, y=w476) -> (x-y=w477:dbl)
        n375 = In Range and Coerce(upper limit=w481, x=w484, lower limit=w480) -> (In Range?=w474:bool)  [unwired: 1 out]
        n376 = In Range and Coerce(upper limit=w478, x=w483, lower limit=w477) -> (In Range?=w473:bool)  [unwired: 1 out]
        n377 = And(x=w474, y=w473) -> (x .and. y?=w472:bool)
        n378 = Not(x=w472) -> (.not. x?=w471:bool)
        n379 = call "ELAPSED TIMER VI.vi"("TARGET"=60.0, "RESET"=w471, "PAUSE"=FALSE) -> ("ELAPSED INDICATION"=w468:bool)  [unwired: 6 in, 2 out]
        n380 = case shown="True" w468 {
          tunnel: w468 -> [_ w487]
          tunnel: [Auto_Start_enum."Maintain Stage" ("Enum - Selector") w486] -> w466
          frame False {
          }
          frame True {
            n381 = stacked-sequence {
              tunnel: w487 -> [_ _ _ _ _]
              tunnel: [_ _ _ _ Auto_Start_enum."Start Stage" ("Enum - Selector")] -> w486
              frame #0 {
                n382 = local read "EVENT LOG"() -> (w489:string)
                n383 = call "Event Log.vi"("Content"="Humidity and temperature set point has stabilized.", "EVENT LOG"=w489) -> ("EVENT LOG"=w490:string)  [unwired: 8 in, 1 out]
                n384 = local write "EVENT LOG"(w490) -> ()
              }
              frame #1 {
                n385 = Wait (ms)(milliseconds to wait=u32 100) -> ()  [unwired: 1 out]
              }
              frame #2 {
                n386 = local read "EVENT LOG"() -> (w493:string)
                n387 = call "Event Log.vi"("Content"="Auto Test Started", "EVENT LOG"=w493) -> ("EVENT LOG"=w494:string)  [unwired: 8 in, 1 out]
                n388 = local write "EVENT LOG"(w494) -> ()
              }
              frame #3 {
                w495 = TRUE ("RUN")
                n389 = local write "RUN"(w495) -> ()
                "Auto Start Temp" <- w495
              }
              frame #4 {
              }
            }
          }
        }
        n390 = local read "Auto Start Test"() -> (w465:bool)
        n391 = Not(x=w465) -> (.not. x?=w464:bool)
        n392 = Select(t=Auto_Start_enum."close", s=w464, f=w466) -> (s? t:f=w467:T11)
      }
      frame "Start Stage" {
        w497 = TRUE ("PAUSE")
        n393 = local read "Auto Start Test"() -> (w502:bool)
        n394 = Not(x=w502) -> (.not. x?=w501:bool)
        n395 = Select(t=Auto_Start_enum."close" ("Enum - Selector"), s=w501, f=Auto_Start_enum."Start Stage" ("Enum - Selector")) -> (s? t:f=w498:T11)
        n396 = call "ELAPSED TIMER VI.vi"("RESET"=w497, "PAUSE"=w497) -> ()  [unwired: 7 in, 3 out]
      }
      frame "close" {
        w503 = FALSE ("Heater Button")
        n397 = local write "RUN"(w503) -> ()
        n398 = local write "Heater Button"(w503) -> ()
        n399 = local write "Humidity"(w503) -> ()
        n400 = local write "Auto Start Test"(w503) -> ()
      }
      frame "Exit" {
      }
    }
    n401 = Wait (ms)(milliseconds to wait=u32 100) -> ()  [unwired: 1 out]
    n402 = local read "Quit"() -> (w415:bool)
  }
  n403 = while {
    stop <- w532 stop-if-true
    w515 = errorcluster {"status"=FALSE, "code"=0, "source"=""} ("error in (no error) 3")
    # "this loop is for manual report generation"
    n404 = local read "Confirm Measrurement"() -> (w514:bool)
    n405 = case shown="True" w514 {
      selector: w514 -> [_ w622]
      tunnel: errorcluster {"status"=FALSE, "code"=0, "source"=""} ("error in (no error) 3") -> [_ w623]
      tunnel: [_ w621] -> _
      frame False {
      }
      frame True {
        n406 = stacked-sequence {
          tunnel: w623 -> [_ w656 _]
          tunnel: w622 -> [_ _ w763]
          tunnel: [_ w644 _] -> w621
          frame #0 {
            n407 = String To Path(string="C:\\LAB-IQ\\Image Calibrate v01.dcf") -> (path=w626:path)
            n408 = Open/Create/Replace File ("Open File")(file path (use dialog)=w626) -> (refnum out=w627:refnum<file>)  [unwired: 5 in, 2 out]
            n409 = for {
              N: 4 -> [_]
              tunnel: w627 -> [w633]
              i -> [w629]
              n410 = Read from Text File ("Read File")(file (use dialog)=w633) -> (text=w634:string)  [unwired: 3 in, 3 out]
              n411 = String Subset(string=w634, offset (0)=6, length (rest)=10 ("length (rest)")) -> (substring=w630:string)
              n412 = Fract/Exp String To Number(string=w630) -> (number=w628:dbl)  [unwired: 3 in, 1 out]
              n413 = case shown="3" w629 {
                tunnel: w628 -> [w635 w636 _ w637 _]
                frame 0 {
                  n414 = local write "5x Gain"(w635) -> ()
                }
                frame 1 {
                  n415 = local write "10x Gain"(w636) -> ()
                }
                frame 2 {
                }
                frame 3 {
                  n416 = local write "100x gain"(w637) -> ()
                }
                frame 4, Default {
                }
              }
            }
          }
          frame #1 {
            n417 = local read "TEST STANDARD"() -> (w639:T3)
            n418 = case shown="\"ISO 12156\"" w639 {
              tunnel: ["ASTM D6079" "ISO 12156"] -> w638
              frame "ASTM D6079", Default {
              }
              frame "ISO 12156" {
              }
            }
            n419 = call "IMAGE ANALYSIS.vi"("Enum"=POST_ANALYSIS_ENUM."GET MEASUREMENTS", "error in"=w656) -> ("error out"=w663:errorcluster)  [unwired: 8 in, 1 out]
            n420 = local read "Magnification :"() -> (w649:string)
            n421 = call "Stall Data Flow.vim"("value in"=w663, "milliseconds to wait"=u32 1000) -> ("value out"=w662:errorcluster)  [unwired: 1 out]
            n422 = local read "Test File List :"() -> (w660:string)
            n423 = case shown="\"10x\"" w649 {
              tunnel: [w699 w700] -> w647
              frame "5x", Default {
                n424 = local read "5x Gain"() -> (w699:dbl)
              }
              frame "10x" {
                # "5x"
                n425 = local read "10x Gain"() -> (w700:dbl)
              }
            }
            n426 = call "IMAGE ANALYSIS.vi"("Enum"=POST_ANALYSIS_ENUM."READ", "error in"=w662) -> ("error out"=w659:errorcluster, "data out"=w650:string)  [unwired: 8 in]
            n427 = Match Pattern(string=w650, regular expression="\"type\": ") -> (after substring=w654:string)  [unwired: 1 in, 3 out]
